vi "Set State.vi"(8 "error in (no error)":errorcluster, 9 "Relay 2":bool, 10 "Relay 1":bool, 11 "Dual Relay Bricklet in":refnum<class "Dual Relay Bricklet.lvclass">) -> (0 "error out":errorcluster, 3 "Dual Relay Bricklet out":refnum<class "Dual Relay Bricklet.lvclass">)   [LabVIEW 2011, in "Tinkerforge.lvlib" / "Dual Relay Bricklet.lvclass"]
doc: "This VI sets both relay states."
uses:
  Dual Relay Bricklet.lvclass
  Device/Device.lvclass
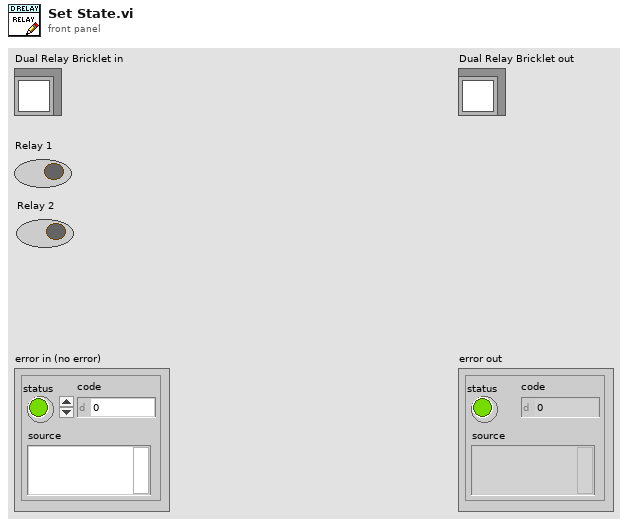
[diagram p1: front panel]
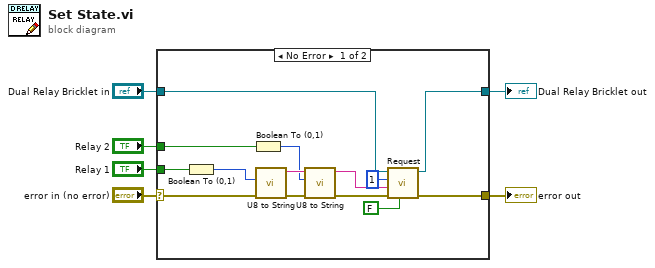
[diagram p0: block diagram]
diagram:
  n1 = case shown="No Error" "error in (no error)" {
    selector: "error in (no error)" -> [w15 w22]
    tunnel: [w16 w22] -> w5
    tunnel: [w19 w21] -> w3
    tunnel: "Dual Relay Bricklet in" -> [w20 w21]
    tunnel: "Relay 2" -> [w10 _]
    tunnel: "Relay 1" -> [w8 _]
    frame No Error {
      n2 = Boolean To (0,1)(Boolean=w8) -> (0, 1=w7:i16)
      n3 = Boolean To (0,1)(Boolean=w10) -> (0, 1=w9:i16)
      n4 = call "U8 to String.vi"("Error In"=w15, "U8"=w7) -> ("Error Out"=w14:errorcluster, "String out"=w11:string)  [unwired: 8 in]
      n5 = call "U8 to String.vi"("Error In"=w14, "U8"=w9, "String in"=w11) -> ("Error Out"=w13:errorcluster, "String out"=w12:string)  [unwired: 7 in]
      n6 = call "Request.vi"("Response"=FALSE, "error in (no error)"=w13, "Data"=w12, "Function ID"=u8 1, "Device in"=w20) -> ("error out"=w16:errorcluster, "Device out"=w19:refnum<class "Dual Relay Bricklet.lvclass">)  [unwired: 2 in, 3 out]
    }
    frame Error {
    }
  }
  "error out" <- w5
  "Dual Relay Bricklet out" <- w3
